vi "Write Boolean.vi"(8 "error in":errorcluster, 9 "value in":bool, 10 "register name":string, 11 "session in":u32) -> (0 "error out":errorcluster, 3 "session out":u32)   [LabVIEW 2018, in "Scalar IO Operations.lvlib"]
uses:
  Scalar IO Operations.lvlib
  NiFpga.dll
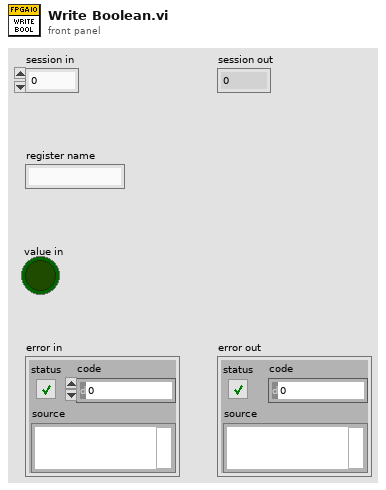
[diagram p1: front panel]
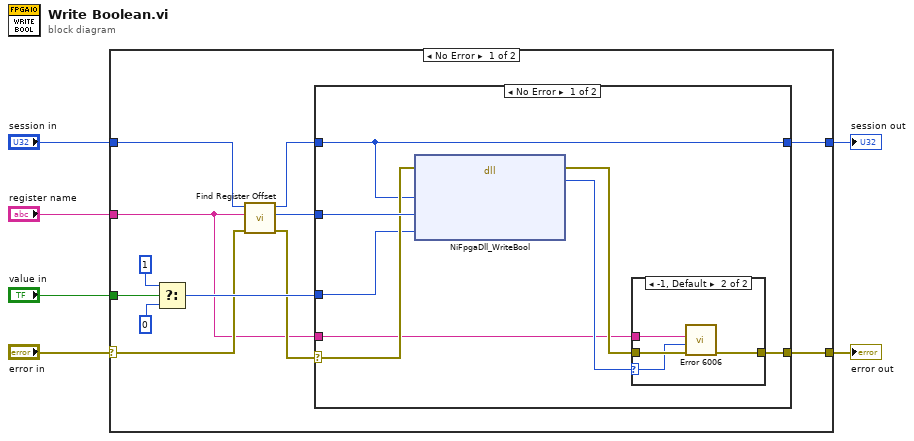
[diagram p0: block diagram]
diagram:
  n1 = case shown="No Error" "error in" {
    selector: "error in" -> [w8 w34]
    tunnel: [w18 w34] -> w6
    tunnel: [w17 w35] -> w5
    tunnel: "value in" -> [w16 _]
    tunnel: "register name" -> [w7 _]
    tunnel: "session in" -> [w12 w35]
    frame No Error {
      n2 = Select(t=u8 1 ("value"), s=w16, f=u8 0) -> (s? t:f=w13:u8)
      n3 = call "Find Register Offset.vi"("error in (no error)"=w8, "register name"=w7, "session in"=w12) -> ("error out"=w11:errorcluster, "resource offset"=w9:u32, "session out"=w10:u32)  [unwired: 6 in]
      n4 = case shown="No Error" w11 {
        selector: w11 -> [w25 w33]
        tunnel: w10 -> [w24 w32]
        tunnel: [w19 w33] -> w18
        tunnel: w9 -> [w26 _]
        tunnel: [w24 w32] -> w17
        tunnel: w13 -> [w23 _]
        tunnel: w7 -> [w20 _]
        frame No Error {
          n5 = dll-call lib="NiFpga.*" fn="NiFpgaDll_WriteBool"(error in=w25, "session"=w24, "offset"=w26, "value"=w23) -> (error out=w21:errorcluster, "status"=w22:i32)  [unwired: 5 in, 1 out]
          n6 = case shown="-1, Default" w22 {
            selector: w22 -> [_ w28]
            tunnel: w21 -> [w27 w29]
            tunnel: [w27 w31] -> w19
            tunnel: w20 -> [_ w30]
            frame 0 {
            }
            frame -1, Default {
              n7 = call "Error 6006.vi"("error in (no error)"=w29, "rio status code"=w28, "register name"=w30) -> ("error out"=w31:errorcluster)  [unwired: 8 in]
            }
          }
        }
        frame Error {
        }
      }
    }
    frame Error {
    }
  }
  "error out" <- w6
  "session out" <- w5
